vi "drive loop.vi"   [LabVIEW 2014]
uses:
  <vilib>/Rock Robotics/Network Tables/SD Write Number.vi
  Global 1.vi
types:
  T1 = typedef "WPI_MotorControlDeviceRef.ctl" = cluster{"DeviceStatus":errorcluster, "Type":T2, "PWM":cluster{"Controller":T3, "PWM Channel":T4, "DeadBand":T5}, "CAN":cluster{"Device Number":u8, "Control Mode":T6, "Semaphore":T7, "Max Vout":dbl, "TalonSRX Control Mode":T8}, "Invert":bool, "TransformRef":T9, "InvTransformRef":T9}
  T2 = typedef "WPI_MotorControlType.ctl" = enum16{"PWM", "CAN", "CANTalonSRX"}
  T3 = typedef "FPGA_TypedefDigitalModule.ctl" = enum16{"Talon 0", "Talon 1", "Talon 2", "Talon 3"}
  T4 = typedef "FPGA_DIOPWMChannel.ctl" = enum8{"PWM 0", "PWM 1", "PWM 2", "PWM 3", "PWM 4", "PWM 5", "PWM 6", "PWM 7", "PWM 8", "PWM 9", "PWM MXP 0", "PWM MXP 1", "PWM MXP 2", "PWM MXP 3", "PWM MXP 4", "PWM MXP 5", "PWM MXP 6", "PWM MXP 7", "PWM MXP 8", "PWM MXP 9", "Invalid"}
  T5 = typedef "WPI_PWMDeadband.ctl" = cluster{"Name":string, "maxPositivePwm":i32, "minPositivePwm":i32, "centerPwm":i32, "maxNegativePwm":i32, "minNegativePwm":i32, "angularRange":u16}
  T6 = typedef "WPI_CANJaguar_ControlMode.ctl" = enum8{"Percent VBus", "Current", "Speed", "Position", "Voltage"}
  T7 = typedef "Semaphore RefNum" = refnum<k1>
  T8 = typedef "WPI_CANTalonSRX_APIControlMode.ctl" = enum8{"Percent VBus", "Speed", "Position", "Slave", "Unchanged / Invalid"}
  T9 = typedef "WPI_PWMTransform_ConPane.ctl" = refnum<vi>
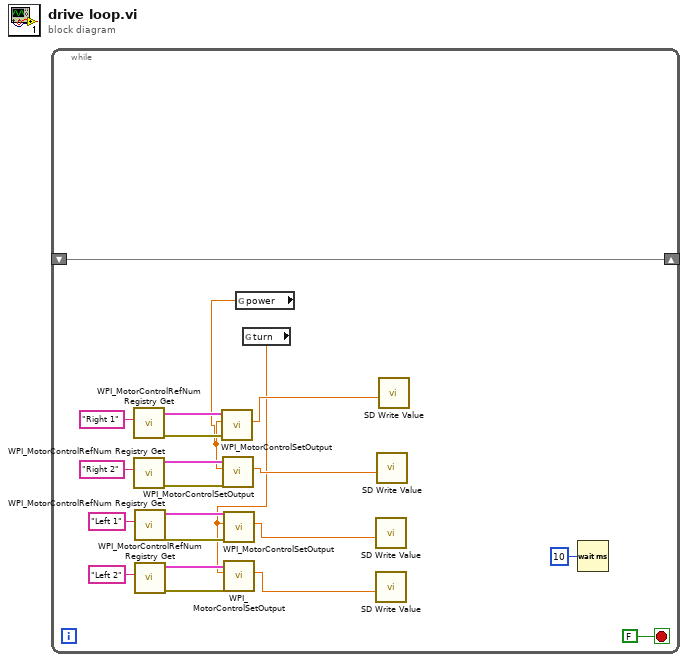
[diagram p0: block diagram]
diagram:
  n1 = while {
    shift-right: [w3] -> _
    shift-left: _ -> [w3]
    stop <- FALSE stop-if-true
    n2 = call <vilib>:"WPI_MotorControlRefNum Registry Get.vi"("refnum name"="Right 1") -> ("error out"=w12:errorcluster, "MotorControlDevRef"=w17:T1)  [unwired: 9 in]
    n3 = call <vilib>:"WPI_MotorControlRefNum Registry Get.vi"("refnum name"="Right 2") -> ("error out"=w11:errorcluster, "MotorControlDevRef"=w16:T1)  [unwired: 9 in]
    n4 = call <vilib>:"WPI_MotorControlRefNum Registry Get.vi"("refnum name"="Left 1") -> ("error out"=w13:errorcluster, "MotorControlDevRef"=w15:T1)  [unwired: 9 in]
    n5 = call <vilib>:"WPI_MotorControlRefNum Registry Get.vi"("refnum name"="Left 2") -> ("error out"=w10:errorcluster, "MotorControlDevRef"=w14:T1)  [unwired: 9 in]
    n6 = global read "Global 1.vi" "power"() -> (w2:dbl)
    n7 = call <vilib>:"WPI_MotorControlSetOutput.vi"("error in (no error)"=w12, "Output"=w2, "MotorControlDevRef"=w17) -> ("Motor Output"=w9:dbl)  [unwired: 6 in, 2 out]
    n8 = call <vilib>:"WPI_MotorControlSetOutput.vi"("error in (no error)"=w11, "Output"=w2, "MotorControlDevRef"=w16) -> ("Motor Output"=w8:dbl)  [unwired: 6 in, 2 out]
    n9 = global read "Global 1.vi" "turn"() -> (w1:dbl)
    n10 = call <vilib>:"WPI_MotorControlSetOutput.vi"("error in (no error)"=w13, "Output"=w1, "MotorControlDevRef"=w15) -> ("Motor Output"=w7:dbl)  [unwired: 6 in, 2 out]
    n11 = call <vilib>:"WPI_MotorControlSetOutput.vi"("error in (no error)"=w10, "Output"=w1, "MotorControlDevRef"=w14) -> ("Motor Output"=w6:dbl)  [unwired: 6 in, 2 out]
    n12 = call-poly <vilib>:"SD Write Value.vi"("Numeric"=w7) -> ()  [unwired: 9 in, 2 out]
    n13 = call-poly <vilib>:"SD Write Value.vi"("Numeric"=w6) -> ()  [unwired: 9 in, 2 out]
    n14 = call-poly <vilib>:"SD Write Value.vi"("Numeric"=w8) -> ()  [unwired: 9 in, 2 out]
    n15 = call-poly <vilib>:"SD Write Value.vi"("Numeric"=w9) -> ()  [unwired: 9 in, 2 out]
    n16 = Wait (ms)(milliseconds to wait=u32 10) -> ()  [unwired: 1 out]
  }
